vi "UsageSetter.vi"   [LabVIEW 2011]
panel:
  # "This VI is only meant to be run from the command line as a built LVEXE.\n\nIt accepts the following arguments following \"--\":\n-target - the name of the target whose usage is being set (required).\n-user - the user setting the target's status (required).\n-in_use - 0 to set as available, 1 to set as in use.  0 is the default."
types:
  T1 = enum32{"invalid app kind", "Development System", "Run Time System", "Student Edition", "Embedded LabVIEW", "Evaluation", "Custom"}
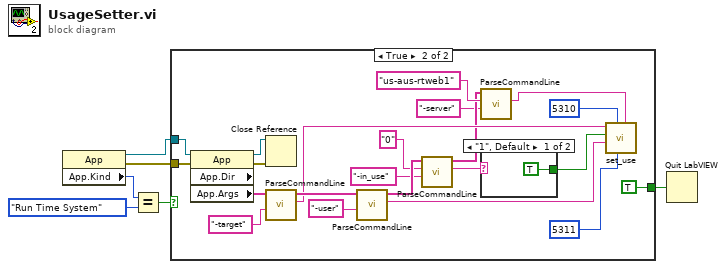
[diagram p0: block diagram]
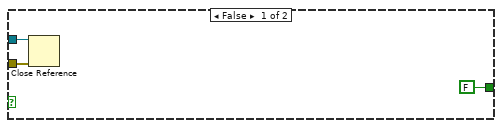
[diagram p2: hidden frame]
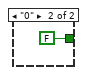
[diagram p3: hidden frame]
diagram:
  n1 = property class="App"() -> (reference out=w5:refnum<vi>, error out=w4:errorcluster, "App.Kind"=w3:T1)  [unwired: 2 in]
  n2 = Equal?(x=w3, y=T1."Run Time System") -> (x = y?=w2:bool)
  n3 = case shown="True" w2 {
    tunnel: w5 -> [w9 w31]
    tunnel: w4 -> [w8 w28]
    tunnel: [FALSE ("quit? (T)") TRUE ("quit? (T)")] -> w1
    frame False {
      n4 = Close Reference(reference=w9, error in (no error)=w8) -> ()  [unwired: 1 out]
    }
    frame True {
      n5 = property class="App" props=["App.Dir", "App.Args"](reference=w31, error in=w28) -> (reference out=w29:refnum<vi>, error out=w30:errorcluster, "App.Args"=w27:string[])  [unwired: 1 out]
      n6 = Close Reference(reference=w29, error in (no error)=w30) -> ()  [unwired: 1 out]
      n7 = call "ParseCommandLine.vi"("Flag"="-target", "App.Args"=w27) -> ("value"=w18:string, "App.Args out"=w25:string[])  [unwired: 7 in, 1 out]
      n8 = call "ParseCommandLine.vi"("Flag"="-user", "App.Args"=w25) -> ("value"=w17:string, "App.Args out"=w24:string[])  [unwired: 7 in, 1 out]
      n9 = call "ParseCommandLine.vi"("Flag"="-in_use", "default value"="0", "App.Args"=w24) -> ("value"=w20:string, "App.Args out"=w12:string[])  [unwired: 6 in, 1 out]
      n10 = call "ParseCommandLine.vi"("Flag"="-server", "default value"="us-aus-rtweb1" ("Remote Server Address"), "App.Args"=w12) -> ("value"=w10:string)  [unwired: 6 in, 2 out]
      n11 = case shown="\"1\", Default" w20 {
        tunnel: [TRUE FALSE] -> w16
        frame "1", Default {
        }
        frame "0" {
        }
      }
      n12 = call "set_use.vi"("Remote Server Address"=w10, "Listen Port"=u16 5311, "Remote Server Port"=u16 5310, "User"=w17, "In Use?"=w16, "Target Name"=w18) -> ()  [unwired: 3 in, 2 out]
    }
  }
  n13 = Quit LabVIEW(quit? (T)=w1) -> ()
